vi "Evaluate.vi"(8 "error in (no error)":errorcluster, 10 "Topic":string, 11 "TopicFilter in":refnum<class "TopicFilter.lvclass">) -> (0 "error out":errorcluster, 1 "Match":bool, 2 "Topic dup":string, 3 "TopicFilter out":refnum<class "TopicFilter.lvclass">)   [LabVIEW 2013, in "MQTT Server.lvlib" / "TopicFilter.lvclass"]
uses:
  TopicFilter.lvclass
  TopicFilter.lvclass/TopicFilter.ctl
panel:
  out "array":string[](array[string])
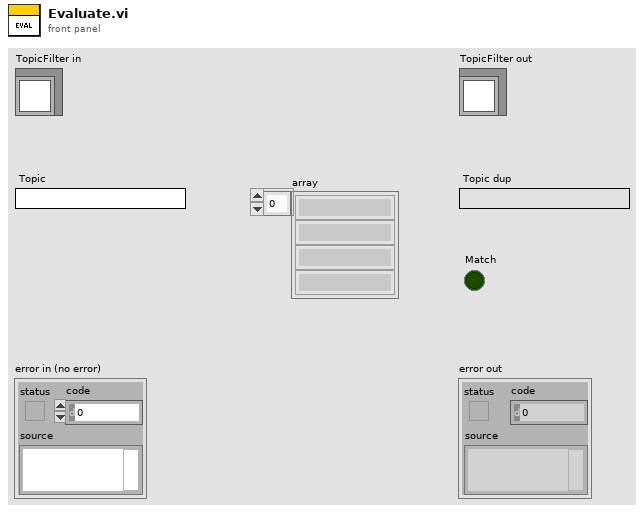
[diagram p1: front panel]
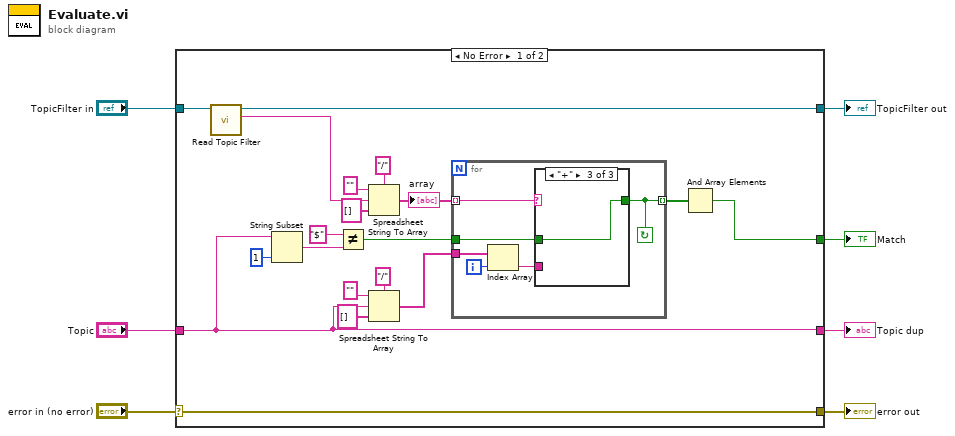
[diagram p0: block diagram]
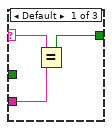
[diagram p2: hidden frame]
diagram:
  n1 = case shown="No Error" "error in (no error)" {
    selector: "error in (no error)" -> [w26 w40]
    tunnel: [w26 w40] -> w6
    tunnel: [w10 w39] -> w4
    tunnel: "TopicFilter in" -> [w11 w39]
    tunnel: "Topic" -> [w8 w38]
    tunnel: [w8 w38] -> w2
    tunnel: [w16 _] -> w1
    frame No Error {
      n2 = call "Read Topic Filter.vi"("TopicFilter in"=w11) -> ("Topic Filter"=w12:string, "TopicFilter out"=w10:refnum<class "TopicFilter.lvclass">)  [unwired: 9 in]
      n3 = String Subset(string=w8, length (rest)=1 ("length (rest)")) -> (substring=w14:string)  [unwired: 1 in]
      n4 = Not Equal?(x="$", y=w14) -> (x != y?=w9:bool)
      n5 = Spreadsheet String To Array(delimiter (Tab)="/", format string="", spreadsheet string=w12, array type (2D Dbl)=string[] []) -> (array=w20:string[])
      "array" <- w20
      n6 = Spreadsheet String To Array(delimiter (Tab)="/", format string="", spreadsheet string=w8, array type (2D Dbl)=string[] []) -> (array=w19:string[])
      n7 = for {
        tunnel: w20 -> [w30] mode=indexing
        tunnel: w19 -> [w32]
        tunnel: [w28] -> w17 mode=indexing
        tunnel: w9 -> [w27]
        i -> [w31]
        stop <- w28 continue-if-true
        n8 = Index Array(array=w32, index=w31) -> (element=w29:string)
        n9 = case shown="\"+\"" w30 {
          selector: w30 -> [w35 _ _]
          tunnel: [w33 w36 w37] -> w28
          tunnel: w29 -> [w34 _ _]
          tunnel: w27 -> [_ w36 w37]
          frame Default {
            n10 = Equal?(x=w35, y=w34) -> (x = y?=w33:bool)
          }
          frame "#" {
          }
          frame "+" {
          }
        }
      }
      n11 = And Array Elements(Boolean array=w17) -> (logical AND=w16:bool)
    }
    frame Error {
    }
  }
  "error out" <- w6
  "TopicFilter out" <- w4
  "Match" <- w1
  "Topic dup" <- w2
